vi "test_codecs.vi"   [LabVIEW 2017]
uses:
  ImageAcquisitionProgram/ImageAcquisitionLibrary/GlobalFrontPanelReferences.vi
  ImageAcquisitionProgram/ImageAcquisitionLibrary/ImageAcquisitionLibrary.lvlib
types:
  T1 = typedef "ImageAcquisitionLibrary.lvlib/References.ctl" = cluster{"Acquire":refnum<vi>, "Rec":refnum<vi>, "Tracking":refnum<vi>, "Settings":refnum<vi>, "Stop":refnum<vi>, "Initialized?":bool, "ImDisplay":refnum<vi>}
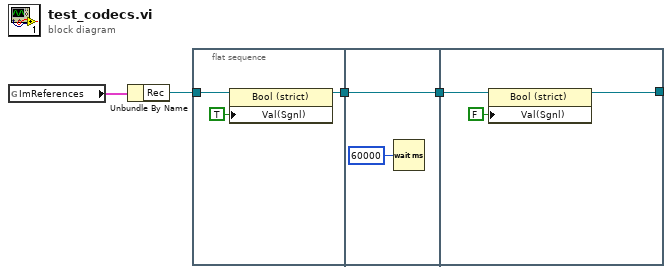
[diagram p0: block diagram]
diagram:
  n1 = global read "GlobalFrontPanelReferences.vi" "ImReferences"() -> (w4:T1)
  n2 = Unbundle By Name(w4) -> ("Rec"=w3:refnum<vi>)
  n3 = flat-sequence {
    tunnel: w3 -> [w7]
    tunnel: [w5] -> w1
    tunnel: [w9] -> w2
    tunnel: w1 -> [w9]
    tunnel: w2 -> [w11]
    tunnel: [w10] -> _
    frame #0 {
      n4 = property class="Bool (strict)"(reference=w7, "Val(Sgnl)"=TRUE ("Value (Signaling)")) -> (reference out=w5:refnum<vi>)  [unwired: 1 in, 1 out]
    }
    frame #1 {
      n5 = Wait (ms)(milliseconds to wait=u32 60000) -> ()  [unwired: 1 out]
    }
    frame #2 {
      n6 = property class="Bool (strict)"(reference=w11, "Val(Sgnl)"=FALSE ("Value (Signaling)")) -> (reference out=w10:refnum<vi>)  [unwired: 1 in, 1 out]
    }
  }
